vi "Schedule.CheckVariantAttributes.vi"(8 "error in (no error)":errorcluster, 11 "Schedule <JSON> In":string) -> (0 "error out":errorcluster, 3 "Schedule <JSON> Out":string)   [LabVIEW 2019, in "ObjectSettings.lvclass"]
uses:
  ObjectSettings.lvclass
  subVIs/typedefs/Schedule Types/Schedule--Constant.ctl
  subVIs/typedefs/Schedule Types/Schedule--Function Generator.ctl
  subVIs/typedefs/Schedule Types/Schedule--Formula.ctl
  subVIs/typedefs/Schedule Types/Schedule--Ramp.ctl
  69576286-dffd-40bf-a4c5-6ac457cf027c.vi
  <vilib>/JDP Science/JSONtext/Variant to JSON Text.vi
  <vilib>/JDP Science/JSONtext/LVClass Serializer/JSONtext LVClass Serializer.lvclass
  <vilib>/JDP Science/JSONtext/JSONtext.lvlib
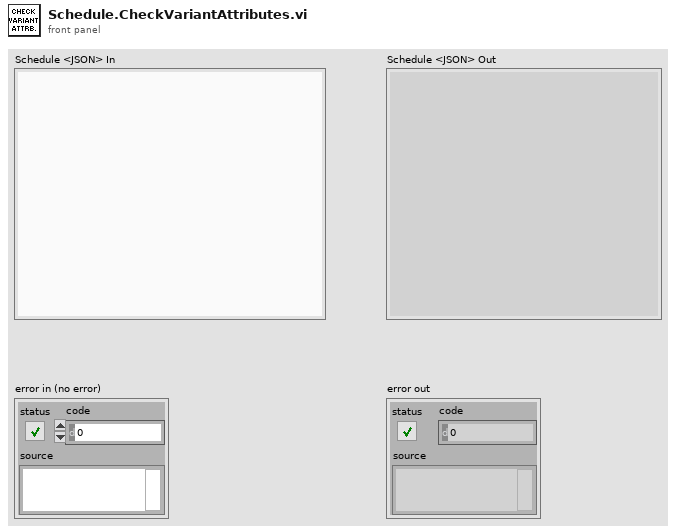
[diagram p1: front panel]
types:
  T1 = typedef "Schedule--Constant.ctl" = cluster{"Value":dbl}
  T2 = typedef "Schedule--Function Generator.ctl" = cluster{"Min Value":dbl, "Max Value":dbl, "Duty Cycle (%)":dbl, "Signal Type":u16, "Cycle Number":dbl, "Phase (degrees)":dbl}
  T3 = typedef "Schedule--Formula.ctl" = cluster{"formula":string, "formula length (nm)":dbl, "formula resolution (nm)":dbl}
  T4 = typedef "Schedule--Ramp.ctl" = cluster{"Start":dbl, "End":dbl}
  T5 = cluster{"Constant":T1, "Fn. Gen":T2, "Formula":T3, "Ramp":T4}
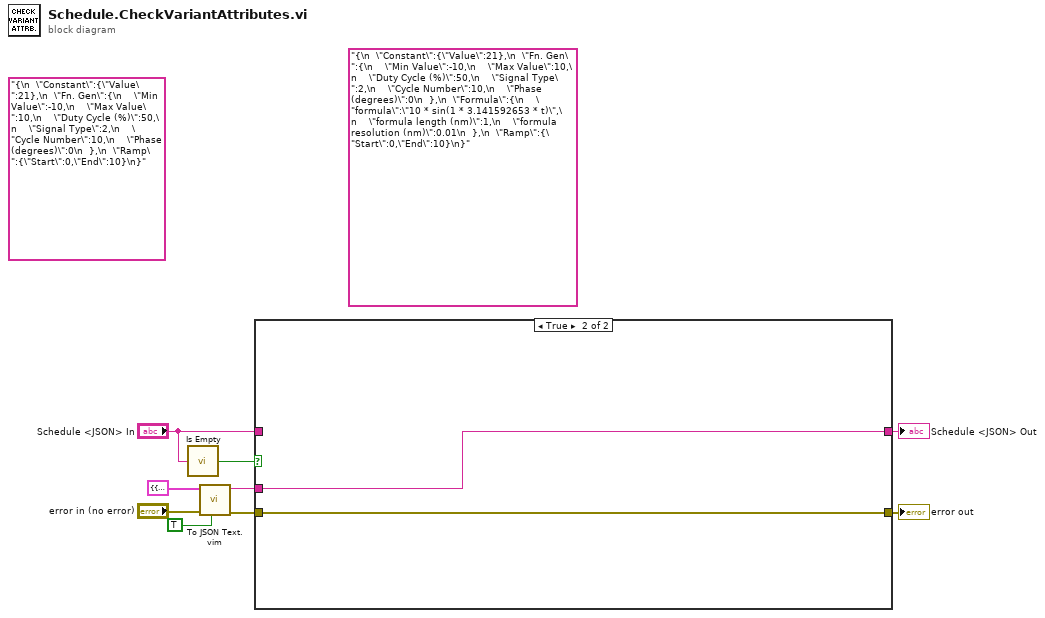
[diagram p0: block diagram]
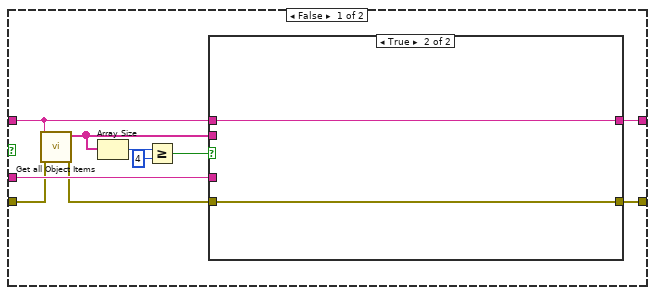
[diagram p2: hidden frame]
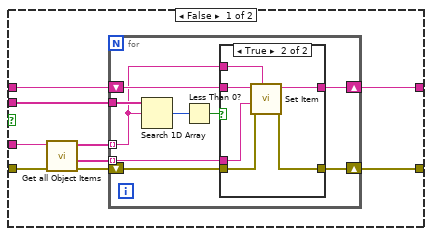
[diagram p3: hidden frame]
diagram:
  (unwired) "{\n  \"Constant\":{\"Value\":21},\n  \"Fn. Gen\":{\n    \"Min Value\":-10,\n    \"Max Value\":10,\n    \"Duty Cycle (%)\":50,\n    \"Signal Type\":2,\n    \"Cycle Number\":10,\n    \"Phase (degrees)\":0\n  },\n  \"Formula\":{\n    \"formula\":\"10 * sin(1 * 3.141592653 * t)\",\n    \"formula length (nm)\":1,\n    \"formula resolution (nm)\":0.01\n  },\n  \"Ramp\":{\"Start\":0,\"End\":10}\n}" ("<JSON> 2")
  (unwired) "{\n  \"Constant\":{\"Value\":21},\n  \"Fn. Gen\":{\n    \"Min Value\":-10,\n    \"Max Value\":10,\n    \"Duty Cycle (%)\":50,\n    \"Signal Type\":2,\n    \"Cycle Number\":10,\n    \"Phase (degrees)\":0\n  },\n  \"Ramp\":{\"Start\":0,\"End\":10}\n}" ("<JSON> 2")
  n1 = call <vilib>:"Is Empty.vi"("JSON"="Schedule <JSON> In") -> ("Empty"=w1:bool)  [unwired: 4 in]
  n2 = call "To JSON Text.vim"("Pretty Print?"=TRUE, "error in (no error)"="error in (no error)", "Anything"=T5 {"Constant"={"Value"=10.0}, "Fn. Gen"={"Min Value"=-10.0, "Max Value"=10.0, "Duty Cycle (%)"=50.0, "Signal Type"=2, "Cycle Number"=10.0, "Phase (degrees)"=0.0}, "Formula"={"formula"="10 * sin(1 * 3.141592653 * t)", "formula length (nm)"=1.0, "formula resolution (nm)"=0.01}, "Ramp"={"Start"=0.0, "End"=10.0}}) -> ("error out"=w5:errorcluster, "<JSON>"=w6:string)  [unwired: 7 in]
  n3 = case shown="True" w1 {
    tunnel: "Schedule <JSON> In" -> [w12 _]
    tunnel: [w15 w49] -> w9
    tunnel: w6 -> [w14 w49]
    tunnel: w5 -> [w10 w48]
    tunnel: [w13 w48] -> w4
    frame False {
      n4 = call <vilib>:"Get all Object Items.vi"("error in (no error)"=w10, "JSON"=w12) -> ("error out"=w11:errorcluster, "Item Names"=w16:string[])  [unwired: 6 in, 2 out]
      n5 = Array Size(array=w16) -> (size(s)=w19:i32)
      n6 = Greater Or Equal?(x=w19, y=4) -> (x >= y?=w17:bool)
      n7 = case shown="True" w17 {
        tunnel: w16 -> [w28 _]
        tunnel: w12 -> [w27 w47]
        tunnel: [w24 w47] -> w15
        tunnel: w14 -> [w23 _]
        tunnel: w11 -> [w22 w46]
        tunnel: [w20 w46] -> w13
        frame False {
          n8 = call <vilib>:"Get all Object Items.vi"("error in (no error)"=w22, "JSON"=w23) -> ("error out"=w21:errorcluster, "<JSON>"=w25:string[], "Item Names"=w26:string[])  [unwired: 6 in, 1 out]
          n9 = for {
            tunnel: w28 -> [w35]
            shift-right: [w36] -> w24
            shift-left: w27 -> [w37]
            tunnel: w26 -> [w31] mode=indexing
            tunnel: w25 -> [w32] mode=indexing
            shift-right: [w29] -> w20
            shift-left: w21 -> [w30]
            n10 = Search 1D Array(1D array=w35, element=w31) -> (index of element=w34:i32)  [unwired: 1 in]
            n11 = Less Than 0?(x=w34) -> (x < 0?=w33:bool)
            n12 = case shown="True" w33 {
              tunnel: w37 -> [w39 w45]
              tunnel: [w39 w44] -> w36
              tunnel: w32 -> [_ w43]
              tunnel: w31 -> [_ w42]
              tunnel: w30 -> [w38 w41]
              tunnel: [w38 w40] -> w29
              frame False {
              }
              frame True {
                n13 = call <vilib>:"Set Item.vi"("$Path or Item Name"=w42, "error in (no error)"=w41, "JSON to Insert"=w43, "JSON"=w45) -> ("error out"=w40:errorcluster, "<JSON>"=w44:string)  [unwired: 4 in, 1 out]
              }
            }
          }
        }
        frame True {
        }
      }
    }
    frame True {
    }
  }
  "error out" <- w4
  "Schedule <JSON> Out" <- w9
